vi "schier save snapshot and single roimasks.vi"() -> ()   [LabVIEW 2014]
uses:
  <vilib>/vision/NI_Vision_Development_Module.lvlib
panel:
  in  "save mask":path=path "C:/Users/Sleep Box/Desktop/rois"
  in  "create mask":bool
  in  "active ROI":dbl
  in  "stop":bool
  in  "load rois":bool
  out "numROIs":i32=96
  out "ROIs":T1={[0, 0, 2592, 1944], [{"Contour Type"=0, "ROI Type"=12, [85, 255, 293, 462, 89840]}, {"Contour Type"=0, "ROI Type"=12, [85, 463, 293, 670, 89840]}, {"Contour Type"=0, "ROI Type"=12, [84, 670, 292, 878, 89840]}, {"Contour Type"=0, "ROI Type"=12, [84, 878, 292, 1085, 89840]}, {"Contour Type"=0, "ROI Type"=12, [84, 1086, 292, 1290, 89840]}, {"Contour Type"=0, "ROI Type"=12, [84, 1294, 292, 1501, 89840]}, {"Contour Type"=0, "ROI Type"=12, [84, 1502, 292, 1708, 89840]}, {"Contour Type"=0, "ROI Type"=12, [83, 1709, 291, 1916, 89840]}, {"Contour Type"=0, "ROI Type"=12, [294, 256, 502, 463, 89840]}, {"Contour Type"=0, "ROI Type"=12, [293, 463, 501, 670, 89840]}, {"Contour Type"=0, "ROI Type"=12, [293, 671, 501, 878, 89840]}, {"Contour Type"=0, "ROI Type"=12, [293, 879, 501, 1086, 89840]}, {"Contour Type"=0, "ROI Type"=12, [293, 1087, 501, 1294, 89840]}, {"Contour Type"=0, "ROI Type"=12, [292, 1294, 500, 1501, 89840]}, {"Contour Type"=0, "ROI Type"=12, [292, 1502, 500, 1709, 89840]}, {"Contour Type"=0, "ROI Type"=12, [292, 1710, 500, 1917, 89840]}, {"Contour Type"=0, "ROI Type"=12, [502, 256, 710, 463, 89840]}, {"Contour Type"=0, "ROI Type"=12, [502, 464, 710, 671, 89840]}, {"Contour Type"=0, "ROI Type"=12, [502, 672, 710, 879, 89840]}, {"Contour Type"=0, "ROI Type"=12, [502, 879, 710, 1086, 89840]}, {"Contour Type"=0, "ROI Type"=12, [501, 1087, 709, 1294, 89840]}, {"Contour Type"=0, "ROI Type"=12, [501, 1295, 709, 1502, 89840]}, {"Contour Type"=0, "ROI Type"=12, [501, 1503, 709, 1710, 89840]}, {"Contour Type"=0, "ROI Type"=12, [501, 1710, 709, 1917, 89840]}, {"Contour Type"=0, "ROI Type"=12, [711, 257, 919, 464, 89840]}, {"Contour Type"=0, "ROI Type"=12, [711, 464, 919, 672, 89840]}, {"Contour Type"=0, "ROI Type"=12, [710, 672, 918, 879, 89840]}, {"Contour Type"=0, "ROI Type"=12, [710, 880, 918, 1087, 89840]}, {"Contour Type"=0, "ROI Type"=12, [710, 1088, 918, 1295, 89840]}, {"Contour Type"=0, "ROI Type"=12, [710, 1296, 918, 1502, 89840]}, {"Contour Type"=0, "ROI Type"=12, [710, 1503, 918, 1710, 89840]}, {"Contour Type"=0, "ROI Type"=12, [709, 1711, 917, 1918, 89840]}, {"Contour Type"=0, "ROI Type"=12, [920, 257, 1128, 464, 89840]}, {"Contour Type"=0, "ROI Type"=12, [919, 465, 1127, 672, 89840]}, {"Contour Type"=0, "ROI Type"=12, [919, 673, 1127, 880, 89840]}, {"Contour Type"=0, "ROI Type"=12, [919, 881, 1127, 1088, 89840]}, {"Contour Type"=0, "ROI Type"=12, [919, 1088, 1127, 1295, 89840]}, {"Contour Type"=0, "ROI Type"=12, [918, 1296, 1126, 1503, 89840]}, {"Contour Type"=0, "ROI Type"=12, [918, 1504, 1126, 1711, 89840]}, {"Contour Type"=0, "ROI Type"=12, [918, 1712, 1126, 1919, 89840]}, {"Contour Type"=0, "ROI Type"=12, [1128, 258, 1336, 465, 89840]}, {"Contour Type"=0, "ROI Type"=12, [1128, 466, 1336, 673, 89840]}, {"Contour Type"=0, "ROI Type"=12, [1128, 673, 1336, 880, 89840]}, {"Contour Type"=0, "ROI Type"=12, [1128, 881, 1336, 1088, 89840]}, {"Contour Type"=0, "ROI Type"=12, [1127, 1089, 1335, 1296, 89840]}, {"Contour Type"=0, "ROI Type"=12, [1127, 1297, 1335, 1504, 89840]}, {"Contour Type"=0, "ROI Type"=12, [1127, 1504, 1335, 1711, 89840]}, {"Contour Type"=0, "ROI Type"=12, [1127, 1712, 1335, 1919, 89840]}, {"Contour Type"=0, "ROI Type"=12, [1337, 258, 1545, 466, 89840]}, {"Contour Type"=0, "ROI Type"=12, [1337, 466, 1545, 673, 89840]}, {"Contour Type"=0, "ROI Type"=12, [1336, 674, 1544, 881, 89840]}, {"Contour Type"=0, "ROI Type"=12, [1336, 882, 1544, 1089, 89840]}, {"Contour Type"=0, "ROI Type"=12, [1336, 1090, 1544, 1296, 89840]}, {"Contour Type"=0, "ROI Type"=12, [1336, 1297, 1544, 1504, 89840]}, {"Contour Type"=0, "ROI Type"=12, [1336, 1505, 1544, 1712, 89840]}, {"Contour Type"=0, "ROI Type"=12, [1335, 1713, 1543, 1920, 89840]}, {"Contour Type"=0, "ROI Type"=12, [1546, 259, 1754, 466, 89840]}, {"Contour Type"=0, "ROI Type"=12, [1545, 467, 1753, 674, 89840]}, {"Contour Type"=0, "ROI Type"=12, [1545, 675, 1753, 882, 89840]}, {"Contour Type"=0, "ROI Type"=12, [1545, 882, 1753, 1089, 89840]}, {"Contour Type"=0, "ROI Type"=12, [1545, 1090, 1753, 1297, 89840]}, {"Contour Type"=0, "ROI Type"=12, [1544, 1298, 1752, 1505, 89840]}, {"Contour Type"=0, "ROI Type"=12, [1544, 1506, 1752, 1713, 89840]}, {"Contour Type"=0, "ROI Type"=12, [1544, 1713, 1752, 1920, 89840]}, {"Contour Type"=0, "ROI Type"=12, [1754, 260, 1962, 467, 89840]}, {"Contour Type"=0, "ROI Type"=12, [1754, 467, 1962, 674, 89840]}, {"Contour Type"=0, "ROI Type"=12, [1754, 675, 1962, 882, 89840]}, {"Contour Type"=0, "ROI Type"=12, [1754, 883, 1962, 1090, 89840]}, {"Contour Type"=0, "ROI Type"=12, [1753, 1091, 1961, 1298, 89840]}, {"Contour Type"=0, "ROI Type"=12, [1753, 1298, 1961, 1505, 89840]}, {"Contour Type"=0, "ROI Type"=12, [1753, 1506, 1961, 1713, 89840]}, {"Contour Type"=0, "ROI Type"=12, [1753, 1714, 1961, 1921, 89840]}, {"Contour Type"=0, "ROI Type"=12, [1963, 260, 2171, 467, 89840]}, {"Contour Type"=0, "ROI Type"=12, [1963, 468, 2171, 675, 89840]}, {"Contour Type"=0, "ROI Type"=12, [1962, 676, 2170, 883, 89840]}, {"Contour Type"=0, "ROI Type"=12, [1962, 884, 2170, 1090, 89840]}, {"Contour Type"=0, "ROI Type"=12, [1962, 1091, 2170, 1298, 89840]}, {"Contour Type"=0, "ROI Type"=12, [1962, 1299, 2170, 1506, 89840]}, {"Contour Type"=0, "ROI Type"=12, [1962, 1507, 2170, 1714, 89840]}, {"Contour Type"=0, "ROI Type"=12, [1961, 1714, 2169, 1922, 89840]}, {"Contour Type"=0, "ROI Type"=12, [2172, 261, 2380, 468, 89840]}, {"Contour Type"=0, "ROI Type"=12, [2171, 469, 2379, 676, 89840]}, {"Contour Type"=0, "ROI Type"=12, [2171, 676, 2379, 883, 89840]}, {"Contour Type"=0, "ROI Type"=12, [2171, 884, 2379, 1091, 89840]}, {"Contour Type"=0, "ROI Type"=12, [2171, 1092, 2379, 1299, 89840]}, {"Contour Type"=0, "ROI Type"=12, [2170, 1300, 2378, 1507, 89840]}, {"Contour Type"=0, "ROI Type"=12, [2170, 1507, 2378, 1714, 89840]}, {"Contour Type"=0, "ROI Type"=12, [2170, 1715, 2378, 1922, 89840]}, {"Contour Type"=0, "ROI Type"=12, [2380, 261, 2588, 468, 89840]}, {"Contour Type"=0, "ROI Type"=12, [2380, 469, 2588, 676, 89840]}, {"Contour Type"=0, "ROI Type"=12, [2380, 677, 2588, 884, 89840]}, {"Contour Type"=0, "ROI Type"=12, [2380, 885, 2588, 1092, 89840]}, {"Contour Type"=0, "ROI Type"=12, [2379, 1092, 2587, 1299, 89840]}, {"Contour Type"=0, "ROI Type"=12, [2379, 1300, 2587, 1507, 89840]}, {"Contour Type"=0, "ROI Type"=12, [2379, 1508, 2587, 1715, 89840]}, {"Contour Type"=0, "ROI Type"=12, [2379, 1716, 2587, 1923, 89840]}]}
  in  "roi data cluster":T1
  in  "Load ROI Data":path=path "C:/Users/Sleep Box/Desktop/rois"
  out "Image":T2(plugin-control)
  in  "Path":path
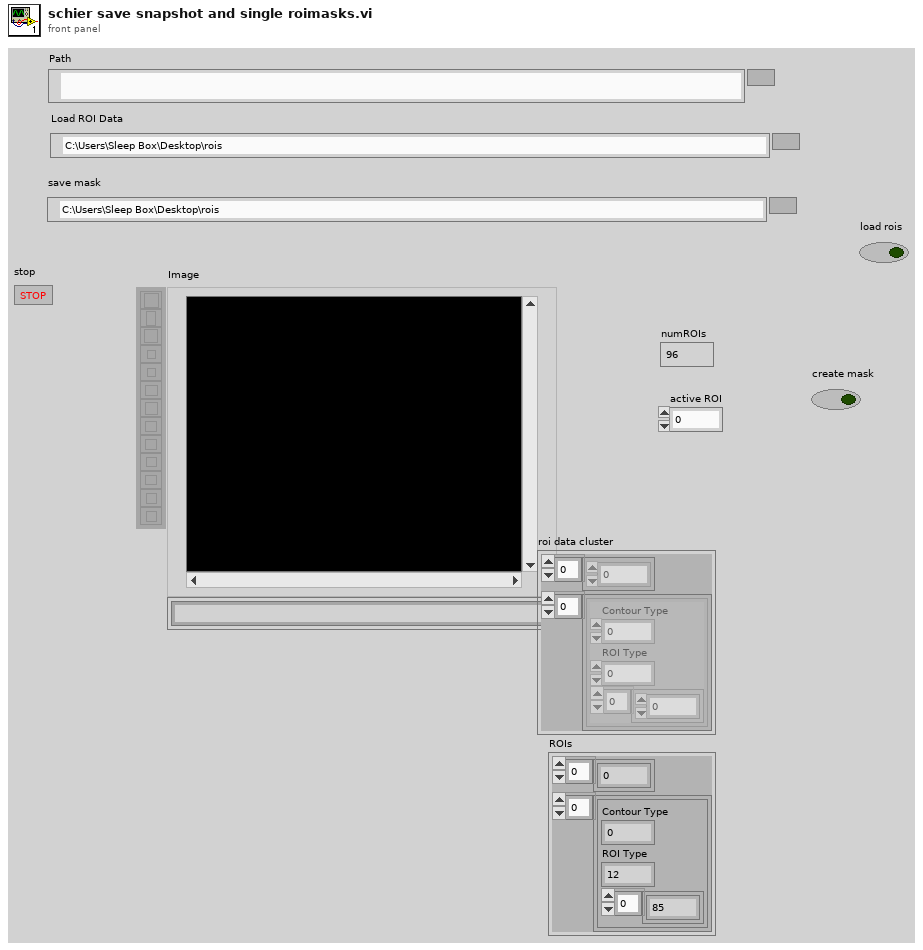
[diagram p1: front panel]
types:
  T1 = cluster{i32[], cluster{"Contour Type":u32, "ROI Type":u32, i32[]}[]}
  T2 = typedef "IMAQ Image.ctl" = refnum<image>
  T3 = cluster{"Contour Type":u32, "ROI Type":u32, i32[]}[]
  T4 = typedef "IMAQ AVI2 Refnum.ctl" = refnum<k20>
  T5 = cluster{"Contour Type":u32, "ROI Type":u32, i32[]}
  T6 = cluster{"Global Rectangle":i32[], "Contours":cluster{"Contour Type":u32, "ROI Type":u32, "Points":i32[]}[]}
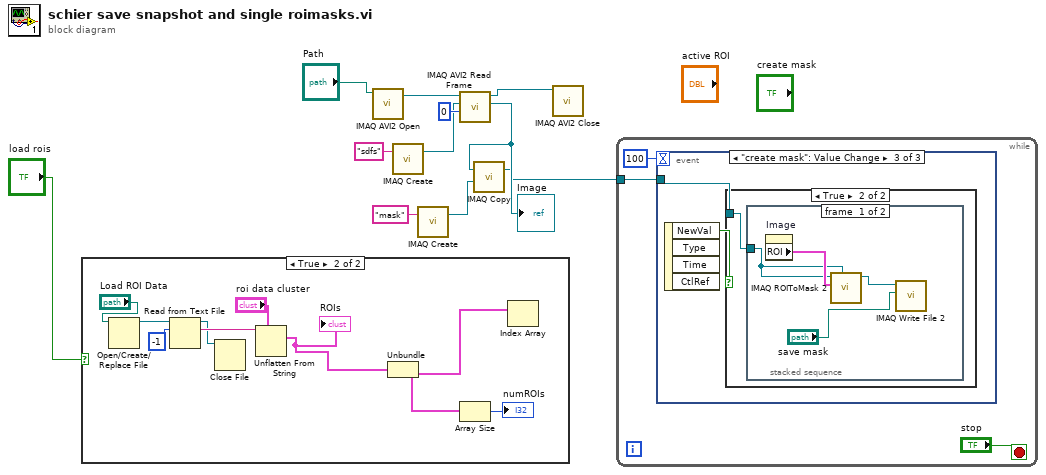
[diagram p0: block diagram]
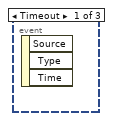
[diagram p2: hidden frame]
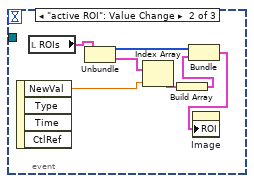
[diagram p3: hidden frame]
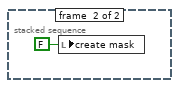
[diagram p5: hidden frame]
diagram:
  n1 = case shown="True" "load rois" {
    frame False {
    }
    frame True {
      n2 = Open/Create/Replace File(file path (use dialog)="Load ROI Data") -> (refnum out=w16:refnum<file>)  [unwired: 5 in, 2 out]
      n3 = Read from Text File(file (use dialog)=w16, count=-1) -> (refnum out=w18:refnum<file>, text=w19:string)  [unwired: 2 in, 2 out]
      n4 = Close File(refnum=w18) -> ()  [unwired: 1 in, 2 out]
      n5 = Unflatten From String(type="roi data cluster", binary string=w19) -> (value=w14:T1)  [unwired: 3 in, 2 out]
      "ROIs" <- w14
      n6 = Unbundle(w14) -> (w12:T3)  [unwired: 1 out]
      n7 = Array Size(array=w12) -> (size(s)=→"numROIs":i32)
      n8 = Index Array(array=w12) -> ()  [unwired: 1 in, 1 out]
    }
  }
  n9 = call "IMAQ AVI2 Open"("AVI File Path"="Path") -> ("AVI Refnum"=w10:T4)  [unwired: 9 in, 1 out]
  n10 = call "IMAQ Create"("Image Name"="sdfs") -> ("New Image"=w7:T2)  [unwired: 4 in, 1 out]
  n11 = call "IMAQ Create"("Image Name"="mask") -> ("New Image"=w2:T2)  [unwired: 4 in, 1 out]
  n12 = call "IMAQ AVI2 Read Frame"("Frame Number"=u32 0, "Image"=w7, "AVI Refnum"=w10) -> ("Image Out"=w3:T2, "AVI Refnum (duplicate)"=w8:T4)  [unwired: 6 in, 1 out]
  "Image" <- w3
  n13 = call "IMAQ Copy"("Image Dst"=w2, "Image Src"=w3) -> ("Image Dst Out"=w1:T2)  [unwired: 4 in, 1 out]
  n14 = call "IMAQ AVI2 Close"("AVI Refnum"=w8) -> ()  [unwired: 10 in, 1 out]
  n15 = while {
    tunnel: w1 -> [w21]
    stop <- "stop" stop-if-true
    n16 = event shown="[2] \"create mask\": Value Change" {
      selector: _ -> [_ _ _]
      dyn-events: _ -> [_ _ _]
      timeout: 100 -> [_ _ _]
      tunnel: w21 -> [_ _ w31]
      event Timeout {
        n17 = event-data() -> ()  [unwired: 1 in, 3 out]
      }
      event "active ROI": Value Change {
        n18 = event-data() -> ("NewVal"=w28:dbl)  [unwired: 1 in, 3 out]
        n19 = local read "ROIs"() -> (w30:T1)
        n20 = Unbundle(w30) -> (w27:i32[], w29:T3)
        n21 = Index Array(array=w29, index=w28) -> (element=w25:T5)
        n22 = Build Array(w25) -> (w24:T3)
        n23 = Bundle(w27, w24) -> (w26:T1)  [unwired: 1 in]
        n24 = property on="Image" class="ImageControl"("ROI"=w26) -> ()  [unwired: 2 in, 2 out]
      }
      event "create mask": Value Change {
        n25 = event-data() -> ("NewVal"=w32:bool)  [unwired: 1 in, 3 out]
        n26 = case shown="True" w32 {
          tunnel: w31 -> [_ w33]
          frame False {
          }
          frame True {
            n27 = stacked-sequence {
              tunnel: w33 -> [w34 _]
              frame #0 {
                n28 = property on="Image" class="ImageControl"() -> ("ROI"=w37:T6)  [unwired: 2 in, 2 out]
                n29 = call "IMAQ ROIToMask 2"("Image Model"=w34, "ROI Descriptor"=w37, "Image"=w34) -> ("Image Out"=w36:T2)  [unwired: 6 in, 2 out]
                n30 = call-poly "IMAQ Write File 2"("File Path"="save mask", "Image"=w36) -> ()  [unwired: 8 in, 2 out]
              }
              frame #1 {
                n31 = local write "create mask"(FALSE ("create mask")) -> ()
              }
            }
          }
        }
      }
    }
  }
